vi "I2C_TEST.vi"() -> ()   [LabVIEW 2014]
uses:
  navX-MXP Library/COMMON/TypeDefs/Data TypeDefs/navX Vector Data.ctl
  navX-MXP Library/COMMON/TypeDefs/Data TypeDefs/navX YPRH Data.ctl
  navX-MXP Library/COMMON/TypeDefs/Data TypeDefs/navX Quaternion Data.ctl
  navX-MXP Library/COMMON/TypeDefs/Data TypeDefs/navX Status Data.ctl
  navX-MXP Library/COMMON/TypeDefs/Value TypeDefs/navX NAVX_OP_STATUS.ctl
  navX-MXP Library/COMMON/TypeDefs/Value TypeDefs/navX NAVX_CAL_STATUS.ctl
  navX-MXP Library/COMMON/TypeDefs/Value TypeDefs/navX NAVX_SENSOR_STATUS.ctl
  <vilib>/Platform/TimedLoop/XDataNode/timing_clust.ctl
  <vilib>/Platform/TimedLoop/XDataNode/nitl_modes.ctl
  <vilib>/Platform/TimedLoop/XDataNode/wakeup.ctl
  <vilib>/platform/TimedLoop/XDataNode/XDataNode.xnode
  navX-MXP Library/navX-MXP IMU.lvlib
  <vilib>/Platform/TimedLoop/XDataNode/XDNodeRunTimeDep.lvlib
panel:
  out "Fused Heading":dbl
  out "Status":T1={"Update Rate Hz"=0, "Accelerometer Full-Scale Range"=0, "Gyro Full-Scale Range"=0, "NAVX_OP_STATUS"=0, "NAVX_CAL_STATUS"=0, "NAVX_SELFTEST_STATUS"=80, "NAVX_SENSOR_STATUS"={"MOVING"=FALSE, "YAW_STABLE"=FALSE, "MAG_DISTURBANCE"=FALSE, "ALTITUDE_VALID"=FALSE, "SEALEVEL_PRESS_SET"=FALSE, "FUSED_HEADING_VALID"=FALSE}} {"NAVX_OP_STATUS" items=["INITIALIZING", "SELFTEST_IN_PROGRESS", "ERROR", "IMU_AUTOCAL_IN_PROGRESS", "NORMAL"]; "NAVX_CAL_STATUS" items=["IMU_CAL_STATE_MASK"=3, "IMU_CAL_INPROGRESS"=0, "IMU_CAL_ACCUMULATE"=1, "IMU_CAL_COMPLETE"=2, "MAG_CAL_COMPLETE"=4, "BARO_CAL_COMPLETE"=8]}
  out "RawMag":T5
  out "RawGyro":T5
  out "RawAccel":T5
  in  "Zero":bool
  out "Quaternion":T6
  out "YPRH":T7
  out "Acceleration":T5
  out "Valid?":bool
  in  "stop":bool
  out "Opened":bool
  in  "Update Rate (4Hz-60Hz)":u8=40
  # "I2C"
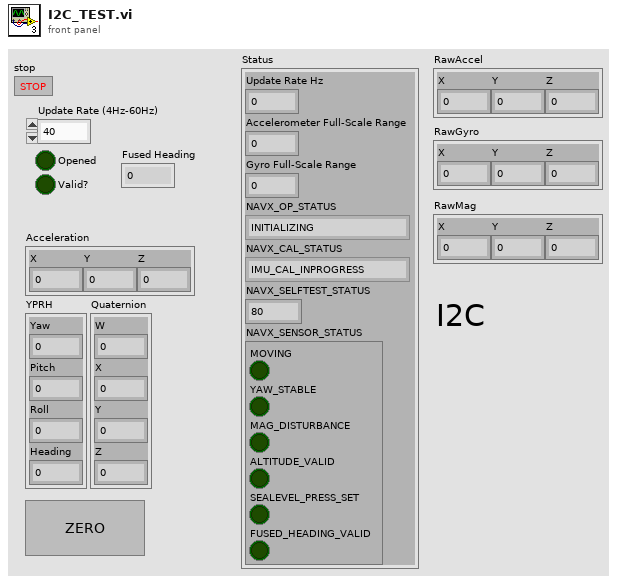
[diagram p1: front panel]
types:
  T1 = typedef "navX-MXP IMU.lvlib/navX Status Data.ctl" = cluster{"Update Rate Hz":u8, "Accelerometer Full-Scale Range":u8, "Gyro Full-Scale Range":u16, "NAVX_OP_STATUS":T2, "NAVX_CAL_STATUS":T3, "NAVX_SELFTEST_STATUS":u8, "NAVX_SENSOR_STATUS":T4}
  T2 = typedef "navX-MXP IMU.lvlib/navX NAVX_OP_STATUS.ctl" = u8
  T3 = typedef "navX-MXP IMU.lvlib/navX NAVX_CAL_STATUS.ctl" = u8
  T4 = typedef "navX-MXP IMU.lvlib/navX NAVX_SENSOR_STATUS.ctl" = cluster{"MOVING":bool, "YAW_STABLE":bool, "MAG_DISTURBANCE":bool, "ALTITUDE_VALID":bool, "SEALEVEL_PRESS_SET":bool, "FUSED_HEADING_VALID":bool}
  T5 = typedef "navX-MXP IMU.lvlib/navX Vector Data.ctl" = cluster{"X":dbl, "Y":dbl, "Z":dbl}
  T6 = typedef "navX-MXP IMU.lvlib/navX Quaternion Data.ctl" = cluster{"W":dbl, "X":dbl, "Y":dbl, "Z":dbl}
  T7 = typedef "navX-MXP IMU.lvlib/navX YPRH Data.ctl" = cluster{"Yaw":dbl, "Pitch":dbl, "Roll":dbl, "Heading":dbl}
  T8 = typedef "navX-MXP IMU.lvlib/navX I2C DevRef.ctl" = cluster{"I2CDevRef":T9, "Board Information":T12, "Status":T1, "Offsets":cluster{"Yaw":dbl, "Quat W":dbl, "Quat X":dbl, "Quat Y":dbl, "Quat Z":dbl}, "Update Rate (4Hz-60Hz)":u8, "refnum name":string, "error":errorcluster}
  T9 = typedef "WPI_I2CDevRef.ctl" = cluster{"DevStatus":errorcluster, "Controller":T10, "Device Address":u8, "Handle":i32, "I2C Bus":T11}
  T10 = typedef "FPGA_TypedefDigitalModule.ctl" = enum16{"Controller 1"}
  T11 = typedef "i2c_bus.ctl" = enum16{"I2C On-Board", "I2C MXP", "Invalid"}
  T12 = typedef "navX-MXP IMU.lvlib/navX Board Information.ctl" = cluster{"WhoAmI (50 | 0x32)":u8, "Board Revision":u8, "Firmware Major Version":u8, "Firmware Minor Version":u8}
  T13 = typedef "XDNodeRunTimeDep.lvlib/timing_clust.ctl" = cluster{"Expected End [f-1]":u64, "Actual End [f-1]":u64, "Finished Late? [f-1]":bool, "Expected End [i-1]":u64, "Actual End [i-1]":u64, "Finished Late? [i-1]":bool, "Expected Start [i]":u64, "Actual Start [i]":u64, "Expected Start [f]":u64, "Actual Start [f]":u64, "Source Name":string, "Structure Name":string, "Period":i64, "Deadline":i64, "Offset":i64, "Start":i64, "Priority":i32, "Timeout":i32, "Mode":T14, "Wakeup Reason":T15, "Error":errorcluster, "Source Type":string, "Secondary Source Type":string, "Global End Time":u64, "Global Start Time":u64, "Frame Duration":u64, "Iteration Duration":u64, "Assigned CPU":i32, "I/O Scan Engine Mode":u32}
  T14 = typedef "XDNodeRunTimeDep.lvlib/nitl_modes.ctl" = enum32{"No Change", "Process missed periods, maintain original phase", "Discard missed periods, maintain original phase", "Process missed periods, ignore original phase", "Discard missed periods, ignore original phase"}
  T15 = typedef "XDNodeRunTimeDep.lvlib/wakeup.ctl" = enum32{"Normal", "Aborted", "Asynchronous wakeup", "Timing source error", "Timed loop error", "Timeout"}
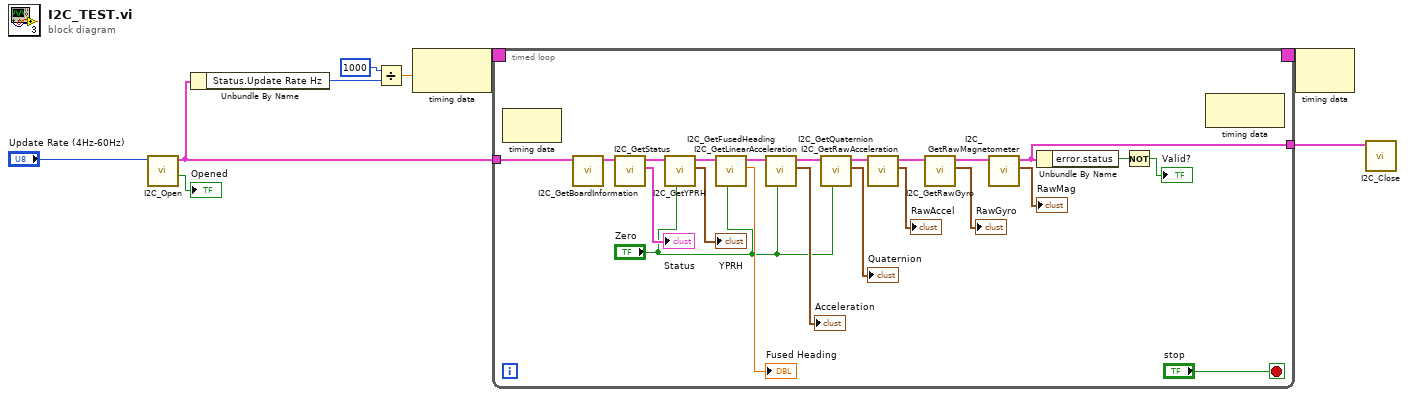
[diagram p0: block diagram]
diagram:
  n1 = call "I2C_Open.vi"("Update Rate (4Hz-60Hz)"="Update Rate (4Hz-60Hz)") -> ("Opened"=→"Opened":bool, "navX DefRef"=w5:T8)  [unwired: 8 in, 1 out]
  n2 = Unbundle By Name(w5) -> ("Status.Update Rate Hz"=w4:u8)
  n3 = Divide(x=1000, y=w4) -> (x/y=w3:dbl)
  n4 = node-c288(w3) -> (w9:T13)
  n5 = timed-loop {
    timing: w9 -> [_]
    timing-out: [_] -> w8
    tunnel: w5 -> [w30]
    tunnel: [w16] -> w7
    stop <- "stop" stop-if-true
    n6 = node-c288() -> ()  [unwired: 1 in, 1 out]
    n7 = call "I2C_GetBoardInformation.vi"("navX DevRef"=w30) -> ("navX DevRef"=w31:T8)  [unwired: 9 in, 1 out]
    n8 = call "I2C_GetStatus.vi"("navX DevRef"=w31) -> ("Status"=→"Status":T1, "navX DefRef"=w29:T8)  [unwired: 9 in]
    n9 = call "I2C_GetYPRH.vi"("Zero"="Zero", "navX DevRef"=w29) -> ("YPRH"=→"YPRH":T7, "navX DevRef"=w28:T8)  [unwired: 8 in]
    n10 = call "I2C_GetFusedHeading.vi"("Zero"="Zero", "navX DevRef"=w28) -> ("Fused Heading"=→"Fused Heading":dbl, "navX DevRef"=w23:T8)  [unwired: 8 in]
    n11 = call "I2C_GetLinearAcceleration.vi"("Zero"="Zero", "navX DevRef"=w23) -> ("Acceleration"=→"Acceleration":T5, "navX DevRef"=w20:T8)  [unwired: 8 in]
    n12 = call "I2C_GetQuaternion.vi"("Zero"="Zero", "navX DevRef"=w20) -> ("Quaternion"=→"Quaternion":T6, "navX DevRef"=w19:T8)  [unwired: 8 in]
    n13 = call "I2C_GetRawAcceleration.vi"("navX DevRef"=w19) -> ("Vector"=→"RawAccel":T5, "navX DevRef"=w18:T8)  [unwired: 9 in]
    n14 = call "I2C_GetRawGyro.vi"("navX DevRef"=w18) -> ("Vector"=→"RawGyro":T5, "navX DevRef"=w17:T8)  [unwired: 9 in]
    n15 = call "I2C_GetRawMagnetometer.vi"("navX DevRef"=w17) -> ("Vector"=→"RawMag":T5, "navX DevRef"=w16:T8)  [unwired: 9 in]
    n16 = Unbundle By Name(w16) -> ("error.status"=w22:bool)
    n17 = Not(x=w22) -> (.not. x?=→"Valid?":bool)
    n18 = node-c288() -> ()  [unwired: 1 in, 1 out]
  }
  n19 = node-c288(w8) -> ()  [unwired: 1 out]
  n20 = call "I2C_Close.vi"("navX DevRef"=w7) -> ()  [unwired: 10 in, 1 out]
